vi "WFPropertiesNULL.vi"() -> (3 "Waveform Properties":T1 {"Ramp (s)" min=0.0; "Fs (Hz)" min=0.0})   [LabVIEW 2009]
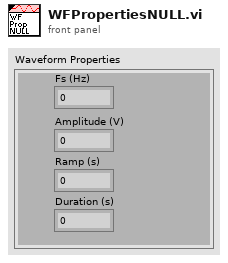
[diagram p1: front panel]
types:
  T1 = cluster{"Fs (Hz)":dbl, "Amplitude (V)":dbl, "Ramp (s)":dbl, "Duration (s)":dbl}
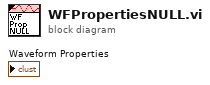
[diagram p0: block diagram]
diagram:
